vi "Zadanie 1.vi"() -> ()   [LabVIEW 2020]
doc: "Use this template to build a producer/consumer design pattern. Use this template when you need to execute a process, such as data analysis, when a data source, such as a triggered acquisition, produces data at an uneven rate and you need to execute the process when the data becomes available."
panel:
  out "Boolean":bool
  out "Zliczenie producent":i32
  out "Liczby":dbl[][](array[numeric])
  out "Obecnie generowana liczba":dbl
  in  "stop":bool
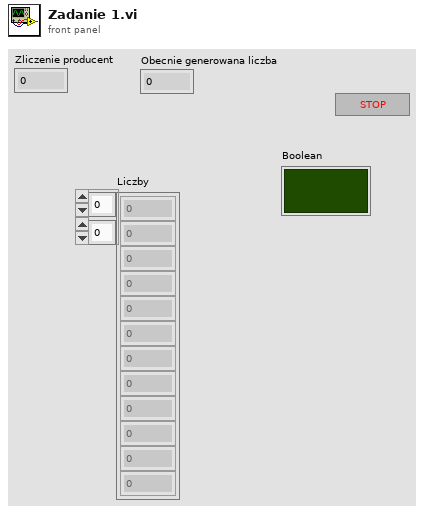
[diagram p1: front panel]
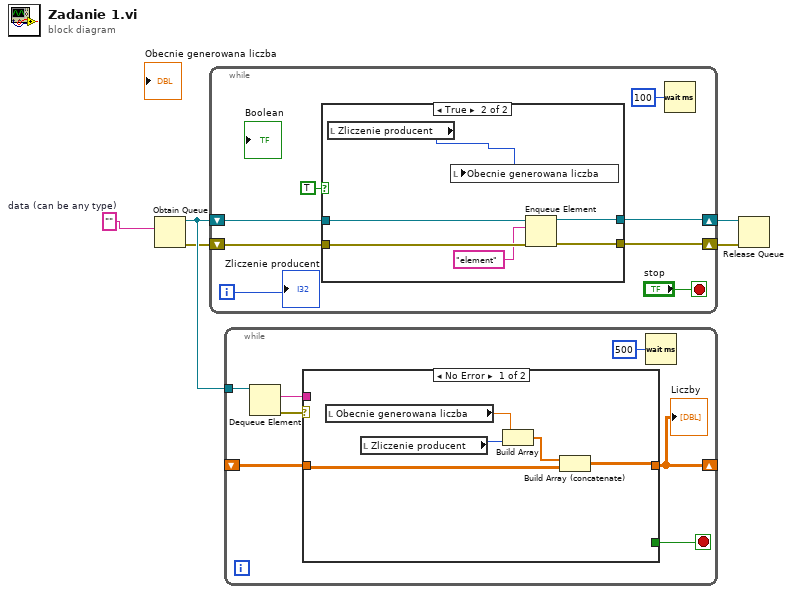
[diagram p0: block diagram]
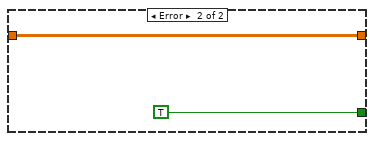
[diagram p2: hidden frame]
diagram:
  w1 = ""  # data (can be any type)
  n1 = Obtain Queue(element data type=w1) -> (queue out=w5:refnum<queue>, error out=w4:errorcluster)  [unwired: 4 in, 1 out]
  n2 = while {
    shift-right: [w9] -> w2
    shift-left: w4 -> [w10]
    shift-right: [w11] -> w3
    shift-left: w5 -> [w12]
    i -> [w6]
    stop <- "stop" stop-if-true
    n3 = case shown="True" TRUE ("Case Constant\n(See Context Help)") {
      tunnel: w12 -> [w15 w21]
      tunnel: [w15 w20] -> w11
      tunnel: w10 -> [w14 w19]
      tunnel: [w14 w18] -> w9
      frame False {
      }
      frame True {
        n4 = local read "Zliczenie producent"() -> (w16:i32)
        n5 = local write "Obecnie generowana liczba"(w16) -> ()
        n6 = Enqueue Element(queue=w21, element="element", error in (no error)=w19) -> (queue out=w20:refnum<queue>, error out=w18:errorcluster)  [unwired: 1 in, 1 out]
      }
    }
    n7 = Wait (ms)(milliseconds to wait=u32 100) -> ()  [unwired: 1 out]
    "Zliczenie producent" <- w6
  }
  n8 = while {
    tunnel: w5 -> [w28]
    shift-right: [w23] -> _
    shift-left: _ -> [w24]
    stop <- w25 stop-if-true
    n9 = Dequeue Element(queue=w28) -> (element=w26:string, error out=w27:errorcluster)  [unwired: 2 in, 2 out]
    n10 = case shown="No Error" w27 {
      tunnel: w26 -> [_ _]
      tunnel: [_ TRUE] -> w25
      tunnel: [w30 w34] -> w23
      tunnel: w24 -> [w31 w34]
      frame No Error {
        n11 = local read "Obecnie generowana liczba"() -> (w33:dbl)
        n12 = local read "Zliczenie producent"() -> (w29:i32)
        n13 = Build Array(w33, w29) -> (w32:dbl[])
        n14 = Build Array (concatenate)(w32, w31) -> (w30:dbl[][])
      }
      frame Error {
      }
    }
    "Liczby" <- w23
    n15 = Wait (ms)(milliseconds to wait=u32 500) -> ()  [unwired: 1 out]
  }
  n16 = Release Queue(queue=w3, error in (no error)=w2) -> ()  [unwired: 1 in, 3 out]
